vi "cvt tag to tag bus tag.vi"(11 "CVT Tags":T1[](array[typedef])) -> (3 "TB Tags":refnum<class "tag descriptor.lvclass">[](array[class]))   [LabVIEW 2013, in "CVT configuration.lvclass"]
uses:
  CVT configuration.lvclass
  <vilib>/NI/Current Value Table/Type Defs/Single Tag.ctl
  <vilib>/NI/Current Value Table/Type Defs/Data Types.ctl
  <vilib>/NI/Tag Bus/tag/tag descriptor.lvclass
  <vilib>/NI/Tag Bus/tag/tag descriptor.lvclass/tag descriptor.ctl
  <vilib>/NI/Current Value Table/Current Value Table.lvlib
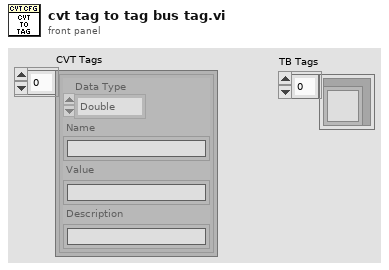
[diagram p1: front panel]
types:
  T1 = typedef "Current Value Table.lvlib/Single Tag.ctl" = cluster{"Data Type":T2, "Name":string, "Value":string, "Description":string}
  T2 = typedef "Current Value Table.lvlib/Data Types.ctl" = enum16{"Double", "Single", "I64", "I32", "I16", "I8", "U64", "U32", "U16", "U8", "String", "Boolean", "Array of U8", "Array of U16", "Array of U32", "Array of U64", "Array of I64", "Array of I32", "Array of I16", "Array of I8", "Array of Double", "Array of Single", "Array of Boolean", "Array of String"}
  T3 = typedef "tag bus.lvlib/tag descriptor.lvclass/Data Type.ctl" = enum16{"Double", "Single", "I64", "I32", "I16", "I8", "U64", "U32", "U16", "U8", "Boolean", "String", "Array of Double", "Array of Single", "Array of I64", "Array of I32", "Array of I16", "Array of I8", "Array of U64", "Array of U32", "Array of U16", "Array of U8", "Array of Boolean", "Array of String"}
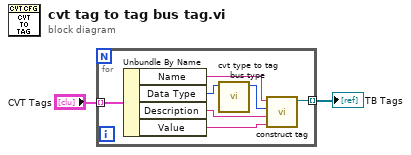
[diagram p0: block diagram]
diagram:
  n1 = for {
    tunnel: "CVT Tags" -> [w9] mode=indexing
    tunnel: [w7] -> w1 mode=indexing
    n2 = Unbundle By Name(w9) -> ("Name"=w6:string, "Data Type"=w8:T2, "Description"=w4:string, "Value"=w3:string)
    n3 = call "cvt type to tag bus type.vi"("cvt type"=w8) -> ("Data Type"=w5:T3)  [unwired: 10 in]
    n4 = call <vilib>:"construct tag.vi"("raw default"=w3, "metadata"=w4, "data type"=w5, "name"=w6) -> ("system tag out"=w7:refnum<class "tag descriptor.lvclass">)  [unwired: 7 in]
  }
  "TB Tags" <- w1
